vi "SA40144D.20210124 BG conductance.vi"() -> ()   [LabVIEW 2020]
uses:
  <userlib>/LevyLab/LV to ITX/Data/Data.lvclass
  <vilib>/Analysis/NI_AALPro.lvlib
panel:
  out "damping 2":dbl
  out "damping":dbl
  in  "parameter bounds":T1={"amp min"=-inf, "amp max"=inf, "damping min"=-inf, "damping max"=inf, "offset min"=0.0, "offset max"=0.0}
  out "G vs t air":T2(graph)
  out "G vs t vacuum":T2(graph)
  out "G vs t heating":T2(graph)
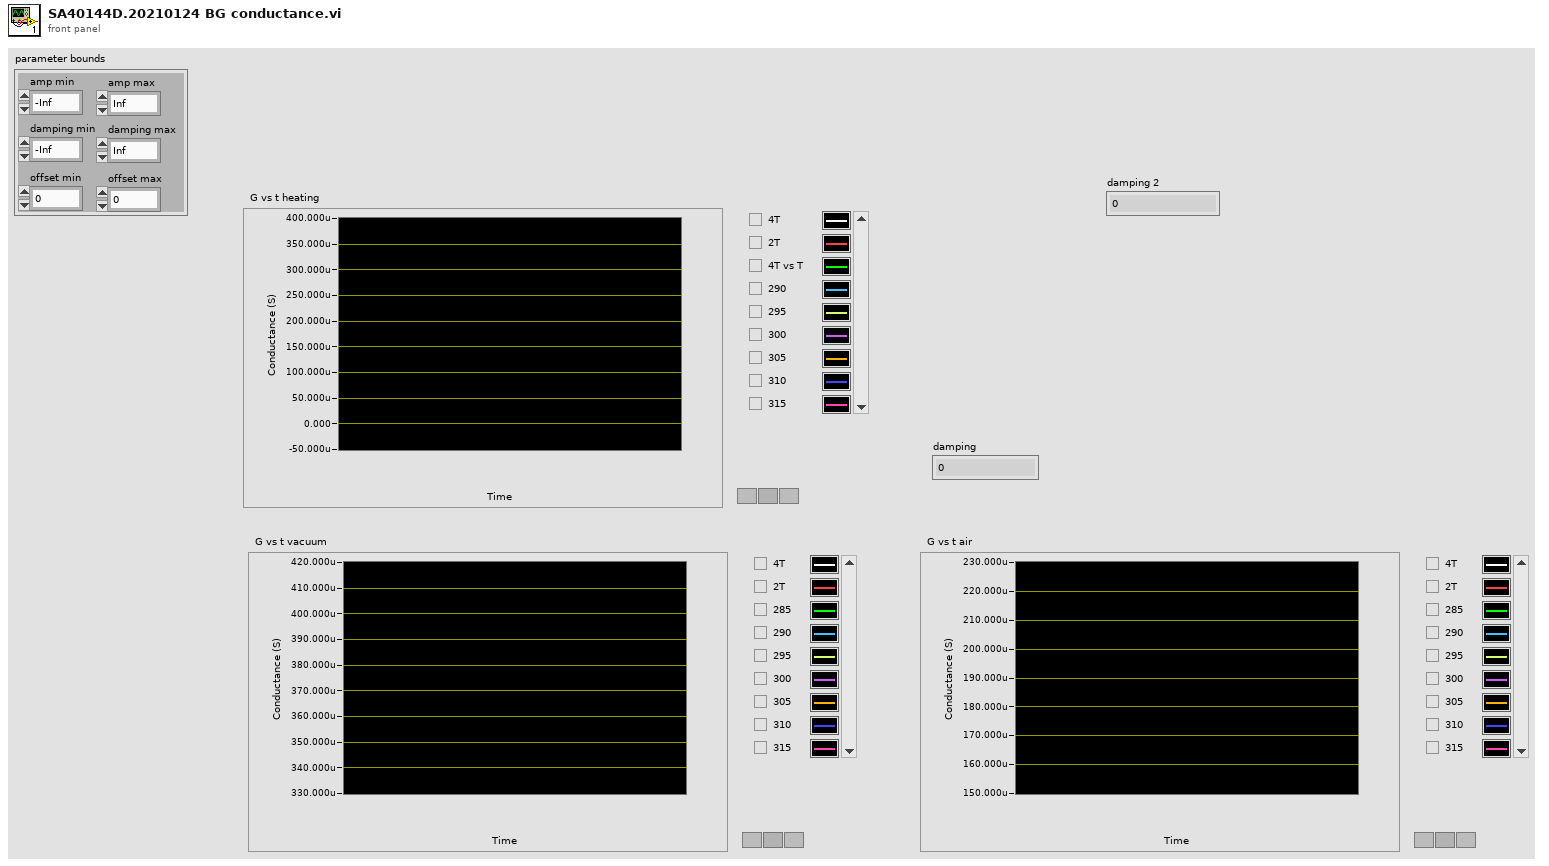
[diagram p1: front panel]
types:
  T1 = cluster{"amp min":dbl, "amp max":dbl, "damping min":dbl, "damping max":dbl, "offset min":dbl, "offset max":dbl}
  T2 = cluster{"Data":dbl[], "Best Exponential Fit":dbl[]}[]
  T3 = typedef "Data.lvclass/Dictionary--cluster.ctl" = cluster{"key":string, "value":variant}
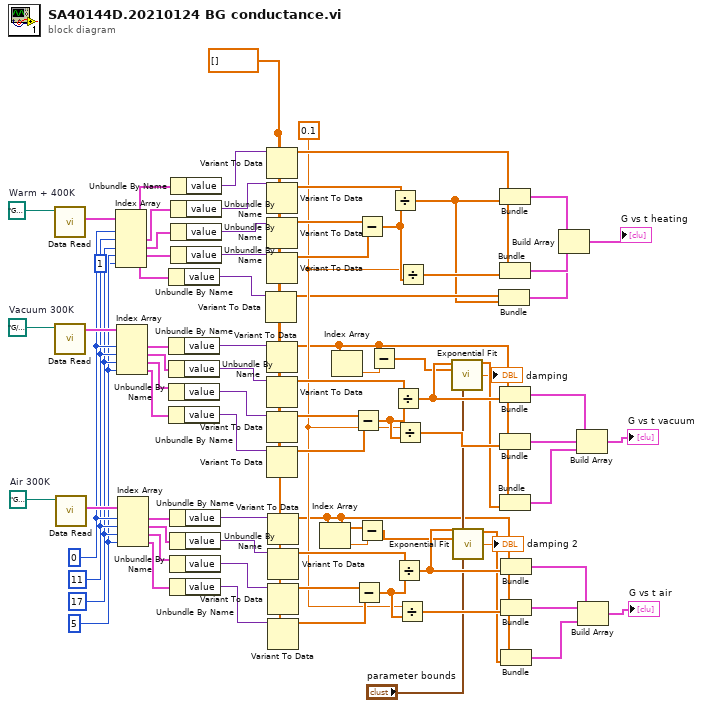
[diagram p0: block diagram]
diagram:
  w45 = path "G:/My Drive/ansom/Data/PPMS 2/SA40144D.20210124/BG Conductance (wrong location/BG Conductance/SA40144D.20210124.000000.dat"  # Air 300K
  w27 = 0.1
  w5 = dbl[] []
  w23 = 5
  w24 = 17
  w25 = 11
  w26 = 0
  w81 = path "G:/My Drive/ansom/Data/PPMS 2/SA40144D.20210124/BG Conductance/SA40144D.20210124.000001.dat"  # Vacuum 300K
  w82 = path "G:/My Drive/ansom/Data/PPMS 2/SA40144D.20210124/BG Conductance/SA40144D.20210124.000000.dat"  # Warm + 400K
  n1 = call <userlib>:"Data Read.vi"("path"=w82) -> ("Data (Dictionary)"=w79:T3[])  [unwired: 7 in, 3 out]
  n2 = call <userlib>:"Data Read.vi"("path"=w81) -> ("Data (Dictionary)"=w80:T3[])  [unwired: 7 in, 3 out]
  n3 = call <userlib>:"Data Read.vi"("path"=w45) -> ("Data (Dictionary)"=w44:T3[])  [unwired: 7 in, 3 out]
  n4 = Index Array(array=w79, index #1=w26, index #2=w25, index #3=w24, index #4=w23, index #5=1 ("index")) -> (element #1=w72:T3, element #2=w73:T3, element #3=w74:T3, element #4=w71:T3, element #5=w6:T3)
  n5 = Index Array(array=w80, index #1=w26, index #2=w25, index #3=w24, index #4=w23) -> (element #1=w78:T3, element #2=w77:T3, element #3=w76:T3, element #4=w75:T3)
  n6 = Index Array(array=w44, index #1=w26, index #2=w25, index #3=w24, index #4=w23) -> (element #1=w43:T3, element #2=w42:T3, element #3=w41:T3, element #4=w40:T3)
  n7 = Unbundle By Name(w6) -> ("value"=w4:variant)
  n8 = Unbundle By Name(w78) -> ("value"=w66:variant)
  n9 = Unbundle By Name(w77) -> ("value"=w65:variant)
  n10 = Unbundle By Name(w76) -> ("value"=w64:variant)
  n11 = Unbundle By Name(w75) -> ("value"=w63:variant)
  n12 = Unbundle By Name(w43) -> ("value"=w39:variant)
  n13 = Unbundle By Name(w42) -> ("value"=w38:variant)
  n14 = Unbundle By Name(w41) -> ("value"=w37:variant)
  n15 = Unbundle By Name(w40) -> ("value"=w36:variant)
  n16 = Unbundle By Name(w72) -> ("value"=w67:variant)
  n17 = Unbundle By Name(w73) -> ("value"=w68:variant)
  n18 = Unbundle By Name(w74) -> ("value"=w69:variant)
  n19 = Unbundle By Name(w71) -> ("value"=w70:variant)
  n20 = Variant To Data(type=w5, Variant=w4) -> (data=w3:dbl[])  [unwired: 1 in, 1 out]
  n21 = Variant To Data(type=w5, Variant=w67) -> (data=w54:dbl[])  [unwired: 1 in, 1 out]
  n22 = Variant To Data(type=w5, Variant=w68) -> (data=w57:dbl[])  [unwired: 1 in, 1 out]
  n23 = Variant To Data(type=w5, Variant=w69) -> (data=w59:dbl[])  [unwired: 1 in, 1 out]
  n24 = Variant To Data(type=w5, Variant=w70) -> (data=w60:dbl[])  [unwired: 1 in, 1 out]
  n25 = Variant To Data(type=w5, Variant=w66) -> (data=w11:dbl[])  [unwired: 1 in, 1 out]
  n26 = Variant To Data(type=w5, Variant=w65) -> (data=w58:dbl[])  [unwired: 1 in, 1 out]
  n27 = Variant To Data(type=w5, Variant=w64) -> (data=w62:dbl[])  [unwired: 1 in, 1 out]
  n28 = Variant To Data(type=w5, Variant=w63) -> (data=w61:dbl[])  [unwired: 1 in, 1 out]
  n29 = Variant To Data(type=w5, Variant=w39) -> (data=w13:dbl[])  [unwired: 1 in, 1 out]
  n30 = Variant To Data(type=w5, Variant=w38) -> (data=w33:dbl[])  [unwired: 1 in, 1 out]
  n31 = Variant To Data(type=w5, Variant=w37) -> (data=w35:dbl[])  [unwired: 1 in, 1 out]
  n32 = Variant To Data(type=w5, Variant=w36) -> (data=w34:dbl[])  [unwired: 1 in, 1 out]
  n33 = Index Array(array=w13) -> (element=w14:dbl)  [unwired: 1 in]
  n34 = Index Array(array=w11) -> (element=w12:dbl)  [unwired: 1 in]
  n35 = Subtract(x=w62, y=w61) -> (x-y=w55:dbl[])
  n36 = Subtract(x=w35, y=w34) -> (x-y=w32:dbl[])
  n37 = Subtract(x=w59, y=w60) -> (x-y=w56:dbl[])
  n38 = Subtract(x=w13, y=w14) -> (x-y=w15:dbl[])
  n39 = Subtract(x=w11, y=w12) -> (x-y=w10:dbl[])
  n40 = Divide(x=w57, y=w56) -> (x/y=w2:dbl[])
  n41 = Divide(x=w58, y=w55) -> (x/y=w19:dbl[])
  n42 = Divide(x=w33, y=w32) -> (x/y=w22:dbl[])
  n43 = Divide(x=w27, y=w55) -> (x/y=w52:dbl[])
  n44 = Divide(x=w27, y=w32) -> (x/y=w31:dbl[])
  n45 = Divide(x=w27, y=w56) -> (x/y=w53:dbl[])
  n46 = call <vilib>:"Exponential Fit.vi"("Y"=w19, "X"=w10, "parameter bounds"="parameter bounds") -> ("Best Exponential Fit"=w18:dbl[], "damping"=→"damping":dbl)  [unwired: 7 in, 4 out]
  n47 = call <vilib>:"Exponential Fit.vi"("Y"=w22, "X"=w15, "parameter bounds"="parameter bounds") -> ("Best Exponential Fit"=w21:dbl[], "damping"=→"damping 2":dbl)  [unwired: 7 in, 4 out]
  n48 = Bundle(w3, w2) -> (w1:cluster{dbl[], dbl[]})  [unwired: 1 in]
  n49 = Bundle(w54, w2) -> (w51:cluster{dbl[], dbl[]})  [unwired: 1 in]
  n50 = Bundle(w54, w53) -> (w50:cluster{dbl[], dbl[]})  [unwired: 1 in]
  n51 = Bundle(w11, w19) -> (w48:cluster{dbl[], dbl[]})  [unwired: 1 in]
  n52 = Bundle(w11, w52) -> (w47:cluster{dbl[], dbl[]})  [unwired: 1 in]
  n53 = Bundle(w11, "Best Exponential Fit"=w18) -> (w17:cluster{dbl[], "Best Exponential Fit":dbl[]})  [unwired: 1 in]
  n54 = Bundle(w13, w22) -> (w30:cluster{dbl[], dbl[]})  [unwired: 1 in]
  n55 = Bundle(w13, w31) -> (w29:cluster{dbl[], dbl[]})  [unwired: 1 in]
  n56 = Bundle(w13, "Best Exponential Fit"=w21) -> (w20:cluster{dbl[], "Best Exponential Fit":dbl[]})  [unwired: 1 in]
  n57 = Build Array(w51, w50, w1) -> (→"G vs t heating":cluster{dbl[], dbl[]}[])
  n58 = Build Array(w48, w47, w17) -> (→"G vs t vacuum":cluster{dbl[], "Best Exponential Fit":dbl[]}[])
  n59 = Build Array(w30, w29, w20) -> (→"G vs t air":cluster{dbl[], "Best Exponential Fit":dbl[]}[])
